vi "setup sub.vi"(7 "Serial port in":refnum<visa-resource-name>) -> (0 "Stepper 1 error out":errorcluster, 1 "Stepper 1 out":T1, 2 "Pin 8 error out":errorcluster, 3 "Pin 8 out":T1, 8 "Stepper 0 error out":errorcluster, 9 "Stepper 0 out":T1, 10 "Pin 2 error out":errorcluster, 11 "Pin 2 out":T1)   [LabVIEW 2018]
uses:
  <vilib>/LabVIEW Interface for Arduino/Type Defs/Arduino Resource.ctl
  <vilib>/LabVIEW Interface for Arduino/Type Defs/Board Type.ctl
  <vilib>/LabVIEW Interface for Arduino/Type Defs/Pin Mode.ctl
  <vilib>/LabVIEW Interface for Arduino/LabVIEW Interface for Arduino.lvlib
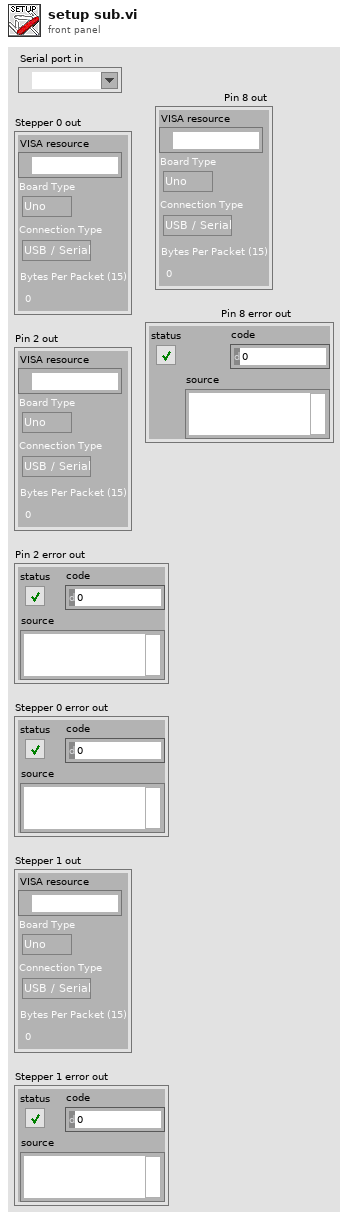
[diagram p1: front panel]
types:
  T1 = typedef "LabVIEW Interface for Arduino.lvlib/Arduino Resource.ctl" = cluster{"VISA resource":refnum<visa-resource-name>, "Board Type":T2, "Connection Type":enum8{"USB / Serial"}, "Bytes Per Packet (15)":u8}
  T2 = typedef "LabVIEW Interface for Arduino.lvlib/Board Type.ctl" = enum16{"Uno", "Dimuelanove w/Atmega 328", "Mega 2560"}
  T3 = typedef "LabVIEW Interface for Arduino.lvlib/Pin Mode.ctl" = enum8{"Input", "Output"}
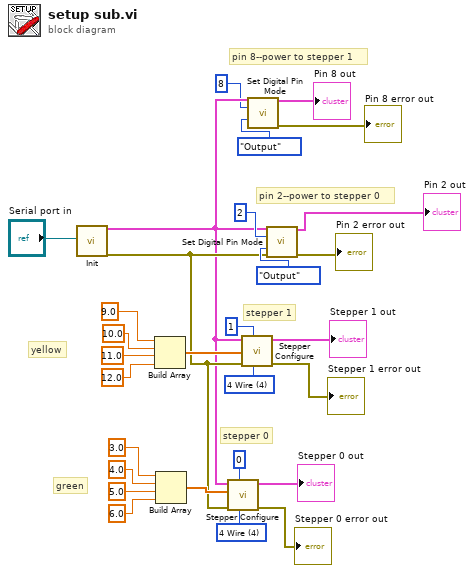
[diagram p0: block diagram]
diagram:
  w29 = u8 4 items=["2 Wire (Pulse & Direction)"=1, "2 Wire"=2, "4 Wire"=4, "EasyDriver"=6, "AF Motor Shield (Stepper 1 & 2 Only)"=5] ("Control Method")
  w16 = u8 4 items=["2 Wire (Pulse & Direction)"=1, "2 Wire"=2, "4 Wire"=4, "EasyDriver"=6, "AF Motor Shield (Stepper 1 & 2 Only)"=5] ("Control Method")
  # "yellow"
  # "green"
  # "pin 8--power to stepper 1"
  # "pin 2--power to stepper 0"
  # "stepper 1"
  # "stepper 0"
  n1 = call <vilib>:"Init.vi"("VISA resource"="Serial port in") -> ("Arduino Resource"=w4:T1, "error out"=w6:errorcluster)  [unwired: 17 in]
  n2 = Build Array(9.0, 10.0, 11.0, 12.0) -> (w24:dbl[])
  n3 = Build Array(3.0, 4.0, 5.0, 6.0) -> (w13:dbl[])
  n4 = call <vilib>:"Stepper Configure.vi"("Control Method"=w16, "Stepper #"=0, "error in"=w6, "Stepper Pins"=w13, "Arduino Resource"=w4) -> ("error out"=→"Stepper 0 error out":errorcluster, "Arduino Resource Out"=→"Stepper 0 out":T1)  [unwired: 5 in]
  n5 = call <vilib>:"Stepper Configure.vi"("Control Method"=w29, "Stepper #"=1, "error in"=w6, "Stepper Pins"=w24, "Arduino Resource"=w4) -> ("error out"=→"Stepper 1 error out":errorcluster, "Arduino Resource Out"=→"Stepper 1 out":T1)  [unwired: 5 in]
  n6 = call <vilib>:"Set Digital Pin Mode.vi"("Arduino Resource"=w4, "Digital I/O Pin"=8, "Pin Mode (Input)"=Pin_Mode."Output") -> ("Arduino Resource"=→"Pin 8 out":T1, "error out"=→"Pin 8 error out":errorcluster)  [unwired: 11 in]
  n7 = call <vilib>:"Set Digital Pin Mode.vi"("Arduino Resource"=w4, "Digital I/O Pin"=2, "Pin Mode (Input)"=Pin_Mode."Output", "error in"=w6) -> ("Arduino Resource"=→"Pin 2 out":T1, "error out"=→"Pin 2 error out":errorcluster)  [unwired: 10 in]
